vi "Color select tree.vi"() -> (2 "Array":u32[](array[numeric]), 3 "Boolean":bool)   [LabVIEW 2020]
uses:
  <vilib>/Rock Robotics/WPI/DriverStation/WPI_DriverStationRobotMode2.ctl
  Robot Global Data.vi
  Globals/Climber_Globals.vi
  Globals/Flywheel_Globals.vi
  Globals/Turret_Globals.vi
  Globals/Cowl_Globals.vi
  Globals/Sensor_Values.vi
  Globals/Autonomous_Globals.vi
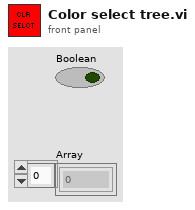
[diagram p1: front panel]
types:
  T1 = typedef "WPI_DriverStationRobotMode2.ctl" = enum16{"Autonomous Disabled", "Autonomous Enabled", "Teleop Disabled", "Teleop Enabled", "Disconnected", "Finish", "Test Disabled", "Test Enabled", "Emergency Stopped"}
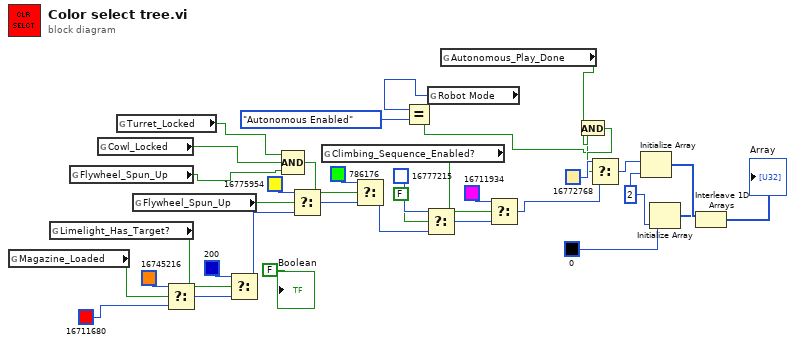
[diagram p0: block diagram]
diagram:
  w3 = 2 ("dimension size")
  n1 = global read "Sensor_Values.vi" "Magazine_Loaded"() -> (w26:bool)
  n2 = global read "Sensor_Values.vi" "Limelight_Has_Target?"() -> (w25:bool)
  n3 = global read "Flywheel_Globals.vi" "Flywheel_Spun_Up"() -> (w35:bool)
  n4 = global read "Cowl_Globals.vi" "Cowl_Locked"() -> (w34:bool)
  n5 = global read "Turret_Globals.vi" "Turret_Locked"() -> (w33:bool)
  n6 = global read "Flywheel_Globals.vi" "Flywheel_Spun_Up"() -> (w16:bool)
  n7 = Select(t=u32 16745216, s=w26, f=u32 16711680) -> (s? t:f=w17:u32)
  n8 = Select(t=u32 200, s=w25, f=w17) -> (s? t:f=w18:u32)
  n9 = Compound Arithmetic op=AND(w33, w34, w35) -> (w15:bool)
  n10 = Select(t=u32 16775954, s=w16, f=w18) -> (s? t:f=w10:u32)
  n11 = global read "Climber_Globals.vi" "Climbing_Sequence_Enabled?"() -> (w13:bool)
  n12 = Select(t=u32 786176, s=w15, f=w10) -> (s? t:f=w7:u32)
  n13 = Select(t=u32 16777215, s=FALSE, f=w7) -> (s? t:f=w8:u32)
  n14 = global read "Robot Global Data.vi" "Robot Mode"() -> (w11:T1)
  n15 = Equal?(x=w11, y=WPI_DriverStationRobotMode2."Autonomous Enabled") -> (x = y?=w27:bool)
  n16 = global read "Autonomous_Globals.vi" "Autonomous_Play_Done"() -> (w28:bool)
  n17 = Select(t=u32 16711934, s=w13, f=w8) -> (s? t:f=w9:u32)
  n18 = And(x=w28, y=w27) -> (x .and. y?=w29:bool)
  n19 = Select(t=u32 16772768, s=w29, f=w9) -> (s? t:f=w31:u32)
  n20 = Initialize Array(w31, w3) -> (w5:u32[])
  n21 = Initialize Array(u32 0, w3) -> (w2:u32[])
  n22 = Interleave 1D Arrays(w5, w2) -> (→"Array":u32[])
  "Boolean" <- FALSE
